vi "Object Tester.vi"() -> ()   [LabVIEW 2025, in "Power Supply.lvlib" / "generic-power-supply.lvclass"]
uses:
  generic-power-supply/generic-power-supply.lvclass
  hardware-selection.ctl
  BK 9202B/BK 9202B.lvclass
  C:/Users/Tyson.Grover/Desktop/Repositories/dqmh-lvoop-template/Libraries/Power Supply/Classes/generic-power-supply/generic-power-supply.lvclass
  <vilib>/Handler Framework/CmdQueue/Enqueue Single.vi
  PSP-603/PSP-603.lvclass
  <vilib>/Handler Framework/Handler Framework.lvlib
panel:
  out "error out":errorcluster
  in  "Tab Control":enum32{"Set Output"}(tab)
  in  "Current":dbl=0.05
  in  "Set Voltage":bool
  in  "Voltage":dbl=10.0
  in  "Set Current":bool
  in  "Output":bool
  out "Voltage [V]":dbl format="%_4g"
  in  "Read Voltage":bool
  in  "Read Current":bool
  out "Current [A]":dbl format="%_4g"
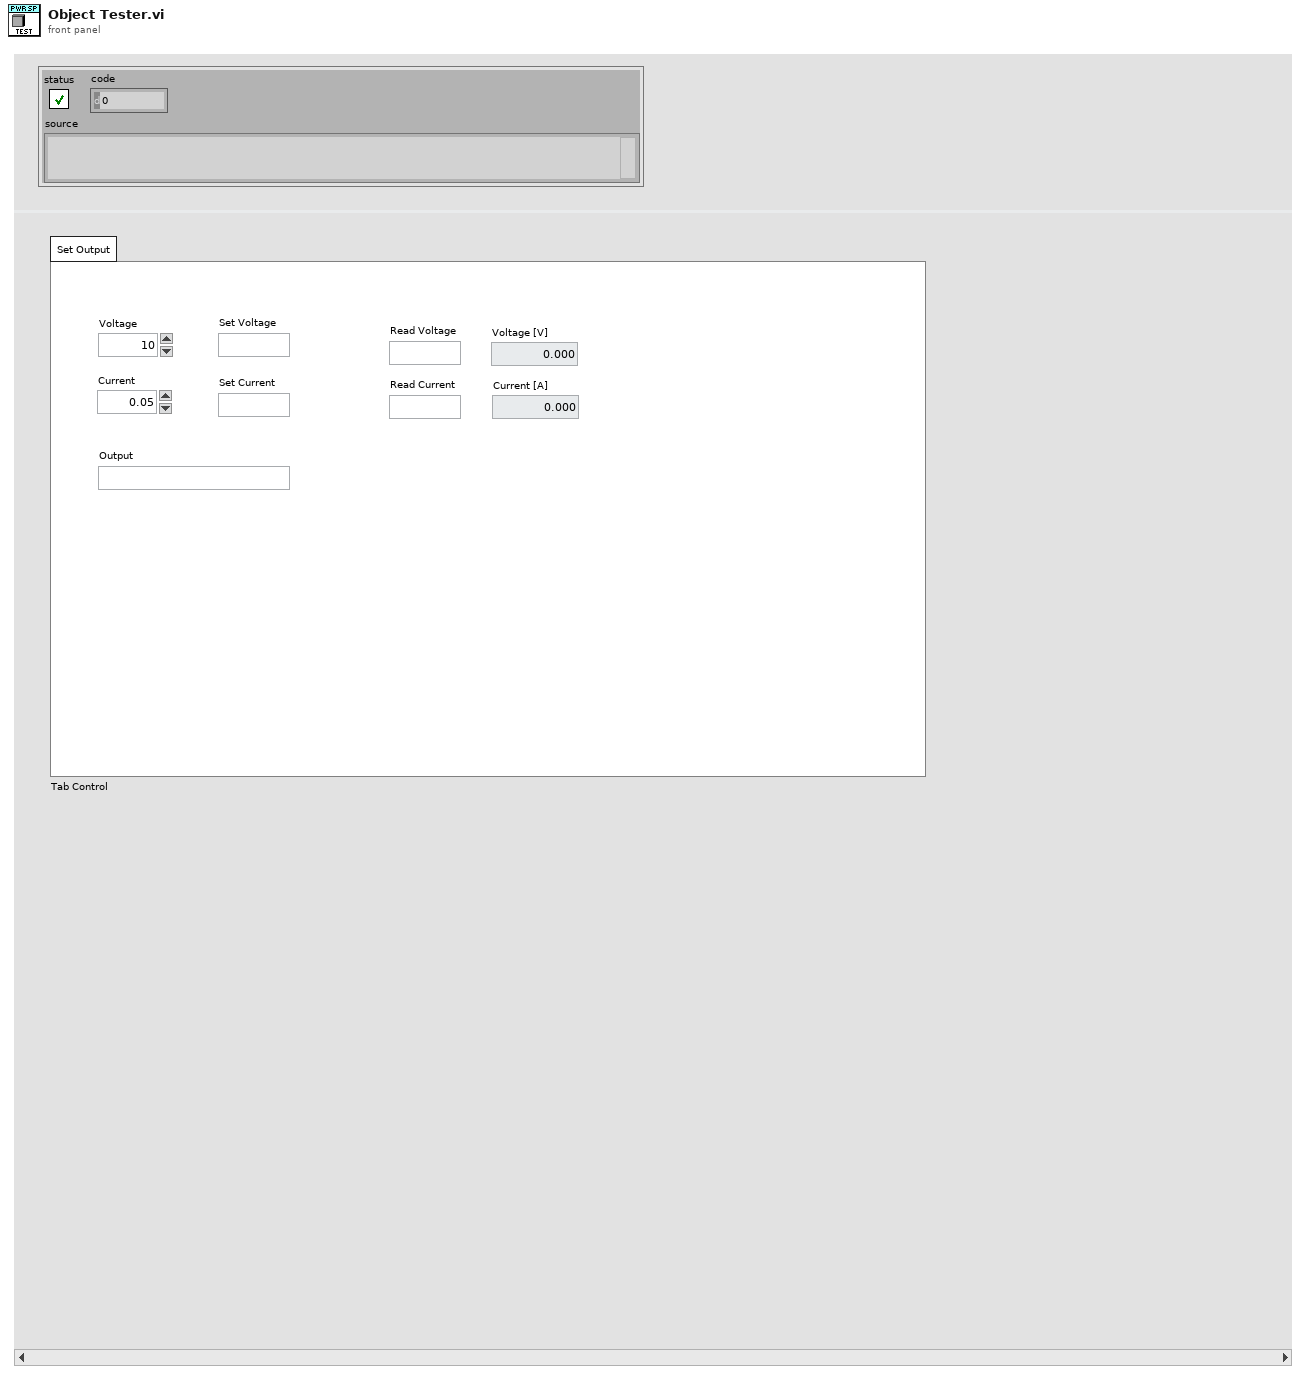
[diagram p1: front panel]
types:
  T1 = typedef "hardware-selection.ctl" = enum16{"Parent", "Simulation", "PSP-603", "BK 9202B"}
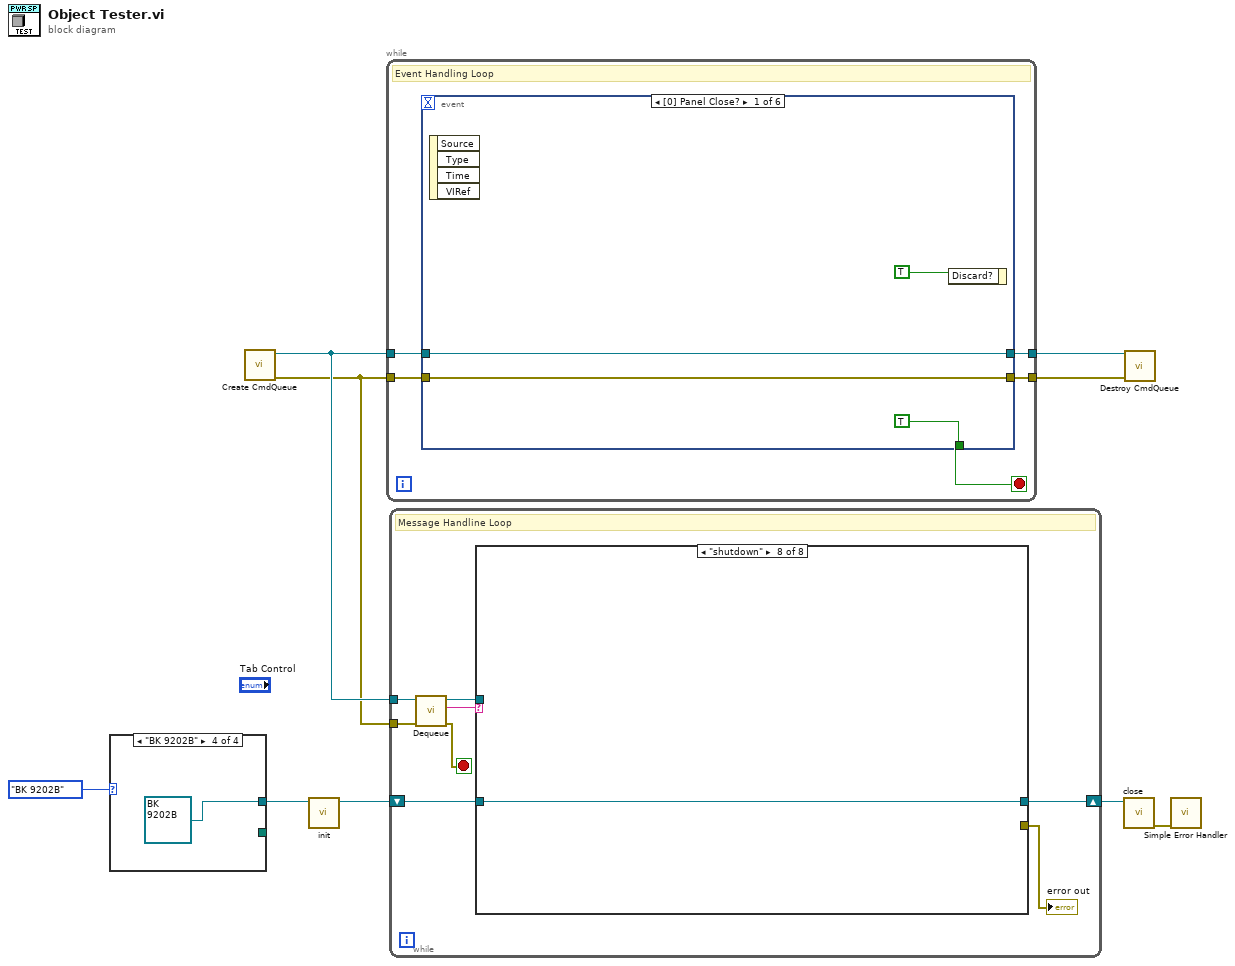
[diagram p0: block diagram]
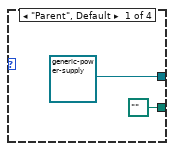
[diagram p2: hidden frame]
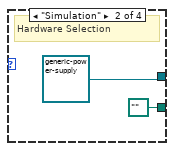
[diagram p3: hidden frame]
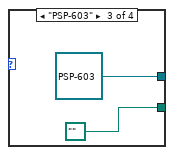
[diagram p4: hidden frame]
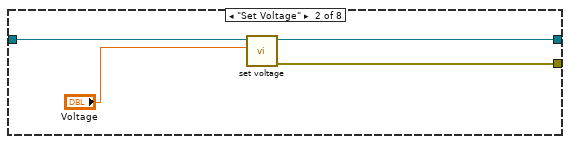
[diagram p6: hidden frame]
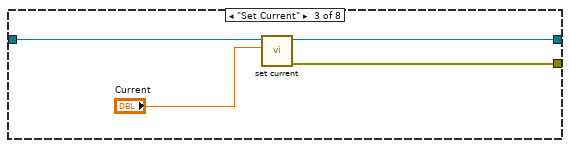
[diagram p7: hidden frame]
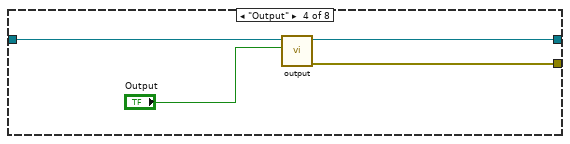
[diagram p8: hidden frame]
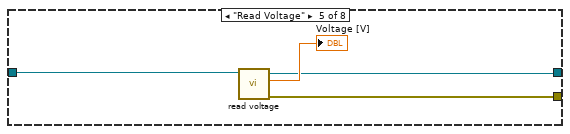
[diagram p9: hidden frame]
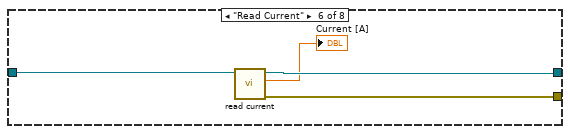
[diagram p10: hidden frame]
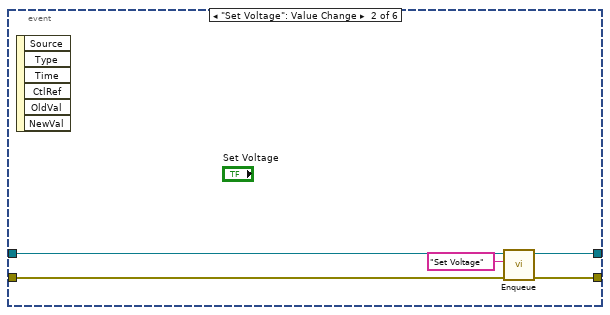
[diagram p12: hidden frame]
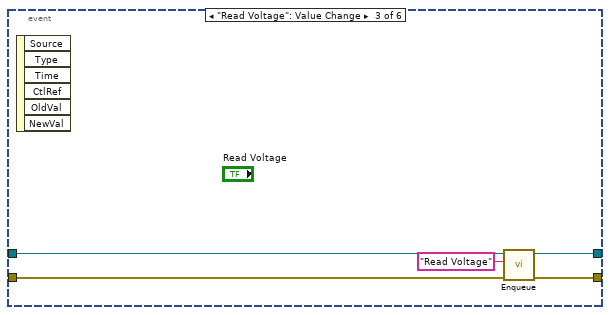
[diagram p13: hidden frame]
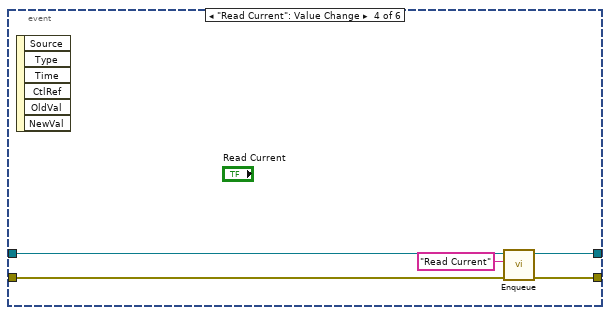
[diagram p14: hidden frame]
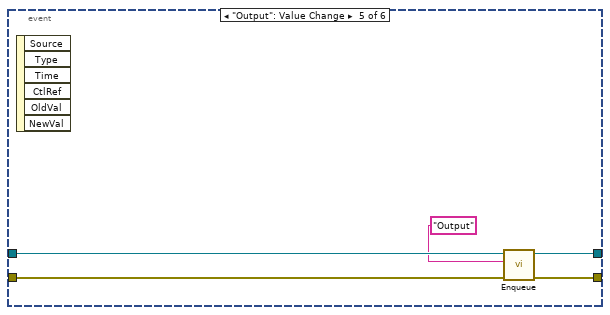
[diagram p15: hidden frame]
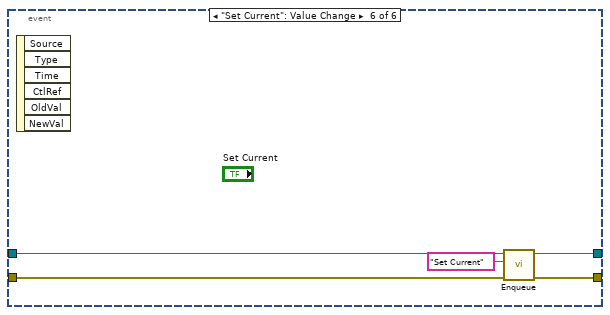
[diagram p16: hidden frame]
diagram:
  n1 = case shown="\"BK 9202B\"" hardware-selection."BK 9202B" {
    tunnel: [path "" ("Path") path "" ("Path") path "" ("Path") _] -> _
    tunnel: [refnum<class "generic-power-supply.lvclass"> refnum ("Power Supply.lvlib:generic-power-supply.lvclass") refnum<class "generic-power-supply.lvclass"> refnum ("Power Supply.lvlib:generic-power-supply.lvclass") refnum<class "PSP-603.lvclass"> refnum ("Power Supply.lvlib:PSP-603.lvclass") refnum<class "BK 9202B.lvclass"> refnum ("Power Supply.lvlib:BK 9202B.lvclass")] -> w4
    frame "Parent", Default {
    }
    frame "Simulation" {
      # "Hardware Selection"
    }
    frame "PSP-603" {
    }
    frame "BK 9202B" {
    }
  }
  n2 = call <vilib>:"Create CmdQueue.vi"() -> ("error out"=w8:errorcluster, "CmdQueue out"=w9:refnum<queue>)  [unwired: 10 in]
  n3 = call-dynamic "init.vi"("generic-power-supply in"=w4) -> ("generic-power-supply out"=w3:refnum<class "generic-power-supply.lvclass">)  [unwired: 9 in, 1 out]
  n4 = while {
    tunnel: w9 -> [w20]
    tunnel: w8 -> [w19]
    tunnel: [w18] -> w7
    tunnel: [w17] -> w6
    stop <- w21 stop-if-true
    # "Event Handling Loop"
    n5 = event shown="[0] Panel Close?" {
      selector: _ -> [_ _ _ _ _ _]
      dyn-events: _ -> [_ _ _ _ _ _]
      timeout: _ -> [_ _ _ _ _ _]
      tunnel: [TRUE _ _ _ _ _] -> w21
      tunnel: w20 -> [w23 w28 w33 w38 w43 w48]
      tunnel: w19 -> [w22 w27 w32 w37 w42 w47]
      tunnel: [w23 w30 w35 w40 w45 w50] -> w18
      tunnel: [w22 w29 w34 w39 w44 w49] -> w17
      event Panel Close? {
        n6 = event-data() -> ()  [unwired: 1 in, 4 out]
        n7 = event-data("Discard?"=TRUE) -> ()  [unwired: 1 in, 1 out]
      }
      event "Set Voltage": Value Change {
        n8 = event-data() -> ()  [unwired: 1 in, 6 out]
        n9 = call-poly <vilib>:"Enqueue.vi"("error in (no error)"=w27, "Command"="Set Voltage", "CmdQueue in"=w28) -> ("error out"=w29:errorcluster, "CmdQueue out"=w30:refnum<queue>)  [unwired: 7 in]
      }
      event "Read Voltage": Value Change {
        n10 = event-data() -> ()  [unwired: 1 in, 6 out]
        n11 = call-poly <vilib>:"Enqueue.vi"("error in (no error)"=w32, "Command"="Read Voltage", "CmdQueue in"=w33) -> ("error out"=w34:errorcluster, "CmdQueue out"=w35:refnum<queue>)  [unwired: 7 in]
      }
      event "Read Current": Value Change {
        n12 = event-data() -> ()  [unwired: 1 in, 6 out]
        n13 = call-poly <vilib>:"Enqueue.vi"("error in (no error)"=w37, "Command"="Read Current", "CmdQueue in"=w38) -> ("error out"=w39:errorcluster, "CmdQueue out"=w40:refnum<queue>)  [unwired: 7 in]
      }
      event "Output": Value Change {
        n14 = event-data() -> ()  [unwired: 1 in, 6 out]
        n15 = call-poly <vilib>:"Enqueue.vi"("error in (no error)"=w42, "Command"="Output", "CmdQueue in"=w43) -> ("error out"=w44:errorcluster, "CmdQueue out"=w45:refnum<queue>)  [unwired: 7 in]
      }
      event "Set Current": Value Change {
        n16 = event-data() -> ()  [unwired: 1 in, 6 out]
        n17 = call-poly <vilib>:"Enqueue.vi"("error in (no error)"=w47, "Command"="Set Current", "CmdQueue in"=w48) -> ("error out"=w49:errorcluster, "CmdQueue out"=w50:refnum<queue>)  [unwired: 7 in]
      }
    }
  }
  n18 = while {
    tunnel: w9 -> [w58]
    tunnel: w8 -> [w57]
    shift-right: [w52] -> w2
    shift-left: w3 -> [w53]
    stop <- w56 stop-if-true
    # "Message Handline Loop"
    n19 = call <vilib>:"Dequeue.vi"("error in (no error)"=w57, "CmdQueue in"=w58) -> ("error out"=w56:errorcluster, "cmd"=w55:string, "CmdQueue out"=w54:refnum<queue>)  [unwired: 5 in, 2 out]
    n20 = case shown="\"shutdown\"" w55 {
      tunnel: w54 -> [_ _ _ _ _ _ _ _]
      tunnel: w53 -> [w59 w63 w67 w71 w75 w79 w80 w81]
      tunnel: [w59 w62 w66 w69 w73 w78 w80 w81] -> w52
      tunnel: [_ w60 w65 w68 w72 w77 _ _] -> w51
      frame Default {
      }
      frame "Set Voltage" {
        n21 = call-dynamic "set voltage.vi"("Voltage"="Voltage", "generic-power-supply in"=w63) -> ("error out"=w60:errorcluster, "generic-power-supply out"=w62:refnum<class "generic-power-supply.lvclass">)  [unwired: 8 in]
      }
      frame "Set Current" {
        n22 = call-dynamic "set current.vi"("Current [A]"="Current", "generic-power-supply in"=w67) -> ("error out"=w65:errorcluster, "generic-power-supply out"=w66:refnum<class "generic-power-supply.lvclass">)  [unwired: 8 in]
      }
      frame "Output" {
        n23 = call-dynamic "output.vi"("Output [on/off]"="Output", "generic-power-supply in"=w71) -> ("error out"=w68:errorcluster, "generic-power-supply out"=w69:refnum<class "generic-power-supply.lvclass">)  [unwired: 8 in]
      }
      frame "Read Voltage" {
        n24 = call-dynamic "read voltage.vi"("generic-power-supply in"=w75) -> ("error out"=w72:errorcluster, "Voltage [V]"=→"Voltage [V]":dbl, "generic-power-supply out"=w73:refnum<class "generic-power-supply.lvclass">)  [unwired: 8 in]
      }
      frame "Read Current" {
        n25 = call-dynamic "read current.vi"("generic-power-supply in"=w79) -> ("error out"=w77:errorcluster, "Current [A]"=→"Current [A]":dbl, "generic-power-supply out"=w78:refnum<class "generic-power-supply.lvclass">)  [unwired: 8 in]
      }
      frame "init" {
      }
      frame "shutdown" {
      }
    }
    "error out" <- w51
  }
  n26 = call-dynamic "close.vi"("generic-power-supply in"=w2) -> ("error out"=w1:errorcluster)  [unwired: 9 in, 1 out]
  n27 = call <vilib>:"Destroy CmdQueue.vi"("error in (no error)"=w6, "CmdQueue in"=w7) -> ()  [unwired: 9 in, 1 out]
  n28 = call <vilib>:"Simple Error Handler.vi"("error in (no error)"=w1) -> ()  [unwired: 4 in, 5 out]
